vi "Thorlabs Translation Stage Module.vi"(7 "Action":T1, 8 "error in (no error)":errorcluster, 9 "Cluster In":T3, 10 "Set/Get":T2, 11 ".NET Refnum in":refnum<k24>) -> (0 "error out":errorcluster, 2 "Cluster out":T3, 3 ".NET Refnum out":refnum<k24>)   [LabVIEW 2017]
uses:
  C:/Users/OCT/Documents/SD-OCT-master/SD-OCT-master/Software/Thorlabs.MotionControl.Controls.dll
  Thorlabs.MotionControl.Controls.dll
  Hardware/Table Stage/Controls/Translation Stage Cluster.ctl
  Controls/Translation Stage Types.ctl
  Controls/Set Get Controls.ctl
  Hardware/Table Stage/Controls/Motion Translation Module Control.ctl
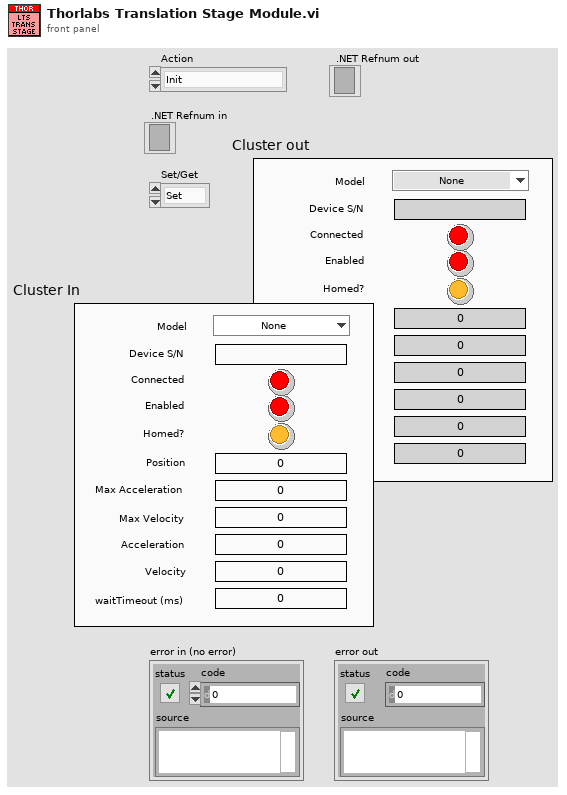
[diagram p1: front panel]
types:
  T1 = typedef "Motion Translation Module Control.ctl" = enum16{"Init", "Home", "Status", "Velocity/Accel", "Position", "Jog", "Stop", "Uninit", "Enable", "Disable"}
  T2 = typedef "Set Get Controls.ctl" = enum16{"Set", "Get"}
  T3 = typedef "Translation Stage Cluster.ctl" = cluster{"Position":dbl, "Is.Enabled?":bool, "Is.Connected?":bool, "Device SN":string, "AccelerationMaximum":dbl, "VelocityMaximum":dbl, "Acceleration":dbl, "Velocity":dbl, "waitTimeout (ms)":i32, "Model":T4, "Is.Homed?":bool}
  T4 = typedef "Translation Stage Types.ctl" = enum16{"None", "Thorlabs LTS", "Thorlabs MLJ"}
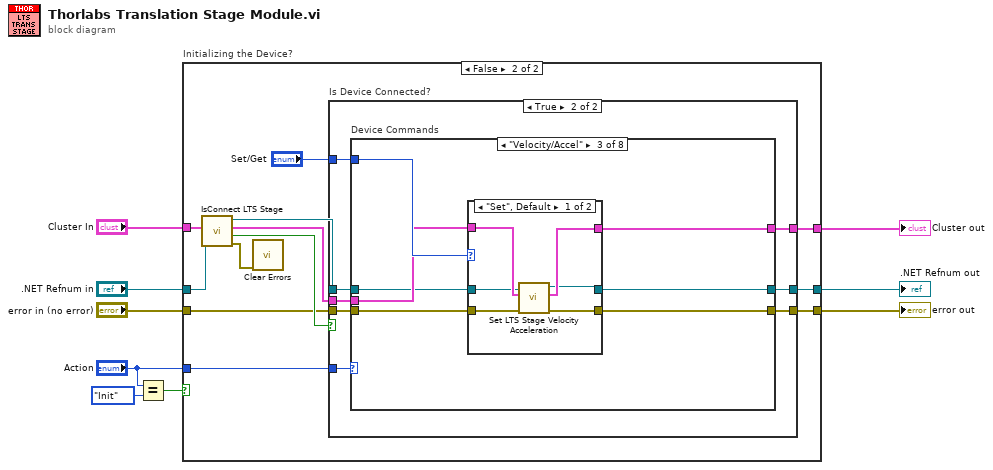
[diagram p0: block diagram]
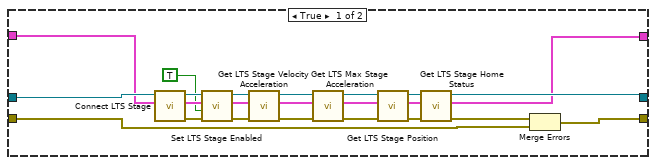
[diagram p2: hidden frame]
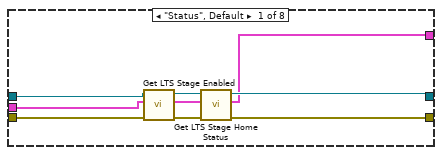
[diagram p4: hidden frame]
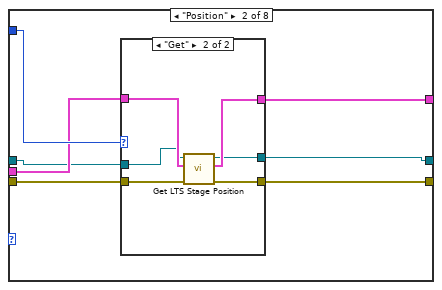
[diagram p5: hidden frame]
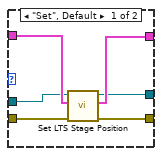
[diagram p6: hidden frame]
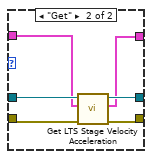
[diagram p7: hidden frame]
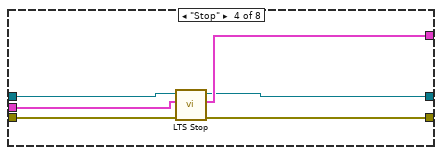
[diagram p8: hidden frame]
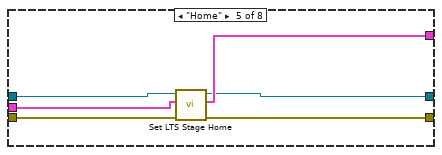
[diagram p9: hidden frame]
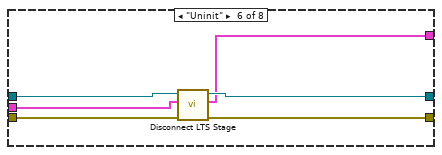
[diagram p10: hidden frame]
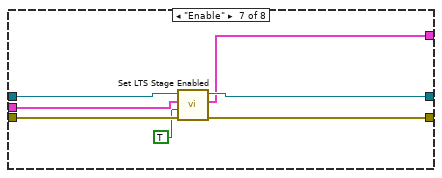
[diagram p11: hidden frame]
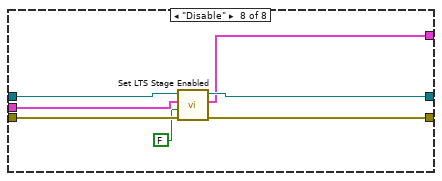
[diagram p12: hidden frame]
diagram:
  n1 = Equal?(x="Action", y=Motion_Translation_Module_Control."Init") -> (x = y?=w1:bool)
  n2 = case "Initializing the Device?" shown="False" w1 {
    tunnel: ".NET Refnum in" -> [w32 w39]
    tunnel: [w19 w44] -> w8
    tunnel: [w18 w43] -> w7
    tunnel: [w16 w42] -> w6
    tunnel: "error in (no error)" -> [w15 w34]
    tunnel: "Cluster In" -> [w31 w36]
    tunnel: "Action" -> [_ w41]
    frame True {
      n3 = call "Connect LTS Stage.vi"("Cluster in"=w31, "LTS Reference In"=w32) -> ("error out"=w30:errorcluster, "Cluster out"=w28:T3, "LTS Reference Out"=w29:refnum<k24>)  [unwired: 6 in, 1 out]
      n4 = call "Set LTS Stage Enabled.vi"("error in (no error)"=w30, "Enable?"=TRUE, "Cluster in"=w28, "LTS Reference In"=w29) -> ("error out"=w27:errorcluster, "Cluster out"=w26:T3, "LTS Reference Out"=w25:refnum<k24>)  [unwired: 5 in]
      n5 = call "Get LTS Stage Velocity Acceleration.vi"("error in (no error)"=w27, "Cluster in"=w26, "LTS Reference In"=w25) -> ("error out"=w24:errorcluster, "Cluster out"=w13:T3, "LTS Reference Out"=w12:refnum<k24>)  [unwired: 5 in, 1 out]
      n6 = call "Get LTS Max Stage Acceleration.vi"("error in (no error)"=w24, "Cluster in"=w13, "LTS Reference In"=w12) -> ("error out"=w14:errorcluster, "Cluster out"=w10:T3, "LTS Reference Out"=w11:refnum<k24>)  [unwired: 4 in, 2 out]
      n7 = call "Get LTS Stage Position.vi"("error in (no error)"=w14, "Cluster in"=w10, "LTS Reference In"=w11) -> ("error out"=w23:errorcluster, "Cluster out"=w21:T3, "LTS Reference Out"=w20:refnum<k24>)  [unwired: 5 in, 1 out]
      n8 = call "Get LTS Stage Home Status.vi"("error in (no error)"=w23, "Cluster in"=w21, "LTS Reference In"=w20) -> ("error out"=w22:errorcluster, "Cluster out"=w18:T3, "LTS Reference Out"=w19:refnum<k24>)  [unwired: 6 in]
      n9 = Merge Errors(w22, w15) -> (w16:errorcluster)
    }
    frame False {
      n10 = call "IsConnect LTS Stage.vi"("Cluster in"=w36, "LTS Reference In"=w39) -> ("error out"=w33:errorcluster, "IsConnected"=w37:bool, "Cluster out"=w35:T3, "LTS Reference Out"=w38:refnum<k24>)  [unwired: 6 in]
      n11 = call <vilib>:"Clear Errors.vi"("error in (no error)"=w33) -> ()  [unwired: 5 in, 2 out]
      n12 = case "Is Device Connected?" shown="True" w37 {
        tunnel: w38 -> [w45 w55]
        tunnel: [w45 w54] -> w44
        tunnel: [w47 w53] -> w43
        tunnel: [w46 w52] -> w42
        tunnel: w34 -> [w46 w51]
        tunnel: "Set/Get" -> [_ w50]
        tunnel: w41 -> [_ w49]
        tunnel: w35 -> [w47 w48]
        frame False {
        }
        frame True {
          n13 = case "Device Commands" shown="\"Velocity/Accel\"" w49 {
            tunnel: w50 -> [_ w71 w90 _ _ _ _ _]
            tunnel: w48 -> [w57 w68 w87 w106 w112 w117 w124 w131]
            tunnel: w51 -> [w58 w70 w89 w108 w114 w120 w127 w134]
            tunnel: [w61 w66 w85 w104 w110 w118 w125 w132] -> w54
            tunnel: [w62 w69 w88 w107 w113 w119 w126 w133] -> w52
            tunnel: [w59 w67 w86 w105 w111 w116 w123 w130] -> w53
            tunnel: w55 -> [w56 w65 w84 w103 w109 w115 w122 w129]
            frame "Status", Default {
              n14 = call "Get LTS Stage Enabled.vi"("error in (no error)"=w58, "Cluster in"=w57, "LTS Reference In"=w56) -> ("error out"=w64:errorcluster, "Cluster out"=w60:T3, "LTS Reference Out"=w63:refnum<k24>)  [unwired: 5 in, 1 out]
              n15 = call "Get LTS Stage Home Status.vi"("error in (no error)"=w64, "Cluster in"=w60, "LTS Reference In"=w63) -> ("error out"=w62:errorcluster, "Cluster out"=w59:T3, "LTS Reference Out"=w61:refnum<k24>)  [unwired: 6 in]
            }
            frame "Position" {
              n16 = case shown="\"Get\"" w71 {
                tunnel: w70 -> [w77 w83]
                tunnel: [w76 w82] -> w69
                tunnel: w68 -> [w75 w81]
                tunnel: [w74 w80] -> w67
                tunnel: w65 -> [w73 w79]
                tunnel: [w72 w78] -> w66
                frame "Set", Default {
                  n17 = call "Set LTS Stage Position.vi"("error in (no error)"=w77, "Cluster in"=w75, "LTS Reference In"=w73) -> ("error out"=w76:errorcluster, "Cluster out"=w74:T3, "LTS Reference Out"=w72:refnum<k24>)  [unwired: 6 in]
                }
                frame "Get" {
                  n18 = call "Get LTS Stage Position.vi"("error in (no error)"=w83, "Cluster in"=w81, "LTS Reference In"=w79) -> ("error out"=w82:errorcluster, "Cluster out"=w80:T3, "LTS Reference Out"=w78:refnum<k24>)  [unwired: 5 in, 1 out]
                }
              }
            }
            frame "Velocity/Accel" {
              n19 = case shown="\"Set\", Default" w90 {
                tunnel: w89 -> [w96 w102]
                tunnel: [w95 w101] -> w88
                tunnel: w87 -> [w93 w98]
                tunnel: [w94 w97] -> w86
                tunnel: w84 -> [w92 w99]
                tunnel: [w91 w100] -> w85
                frame "Set", Default {
                  n20 = call "Set LTS Stage Velocity Acceleration.vi"("error in (no error)"=w96, "Cluster in"=w93, "LTS Reference In"=w92) -> ("error out"=w95:errorcluster, "Cluster out"=w94:T3, "LTS Reference Out"=w91:refnum<k24>)  [unwired: 6 in]
                }
                frame "Get" {
                  n21 = call "Get LTS Stage Velocity Acceleration.vi"("error in (no error)"=w102, "Cluster in"=w98, "LTS Reference In"=w99) -> ("error out"=w101:errorcluster, "Cluster out"=w97:T3, "LTS Reference Out"=w100:refnum<k24>)  [unwired: 5 in, 1 out]
                }
              }
            }
            frame "Stop" {
              n22 = call "LTS Stop.vi"("error in (no error)"=w108, "Cluster in"=w106, "LTS Reference In"=w103) -> ("error out"=w107:errorcluster, "Cluster out"=w105:T3, "LTS Reference Out"=w104:refnum<k24>)  [unwired: 6 in]
            }
            frame "Home" {
              n23 = call "Set LTS Stage Home.vi"("error in (no error)"=w114, "Cluster in"=w112, "LTS Reference In"=w109) -> ("error out"=w113:errorcluster, "Cluster out"=w111:T3, "LTS Reference Out"=w110:refnum<k24>)  [unwired: 6 in]
            }
            frame "Uninit" {
              n24 = call "Disconnect LTS Stage.vi"("error in (no error)"=w120, "Cluster in"=w117, "LTS Reference In"=w115) -> ("error out"=w119:errorcluster, "Cluster out"=w116:T3, "LTS Reference Out"=w118:refnum<k24>)  [unwired: 6 in]
            }
            frame "Enable" {
              n25 = call "Set LTS Stage Enabled.vi"("error in (no error)"=w127, "Enable?"=TRUE, "Cluster in"=w124, "LTS Reference In"=w122) -> ("error out"=w126:errorcluster, "Cluster out"=w123:T3, "LTS Reference Out"=w125:refnum<k24>)  [unwired: 5 in]
            }
            frame "Disable" {
              n26 = call "Set LTS Stage Enabled.vi"("error in (no error)"=w134, "Enable?"=FALSE, "Cluster in"=w131, "LTS Reference In"=w129) -> ("error out"=w133:errorcluster, "Cluster out"=w130:T3, "LTS Reference Out"=w132:refnum<k24>)  [unwired: 5 in]
            }
          }
        }
      }
    }
  }
  ".NET Refnum out" <- w8
  "Cluster out" <- w7
  "error out" <- w6
